vi "Make.vi"(8 "error in (no error)":errorcluster, 11 "Electrical in":refnum<class "Electrical.lvclass">) -> (0 "error out":errorcluster, 3 "Electrical out":refnum<class "Electrical.lvclass">)   [LabVIEW 2014, in "Electrical.lvclass"]
uses:
  Electrical.lvclass
  Paint/Paint.lvclass
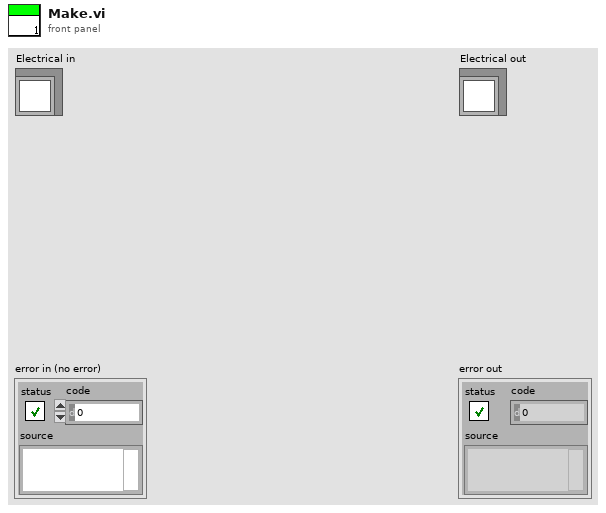
[diagram p1: front panel]
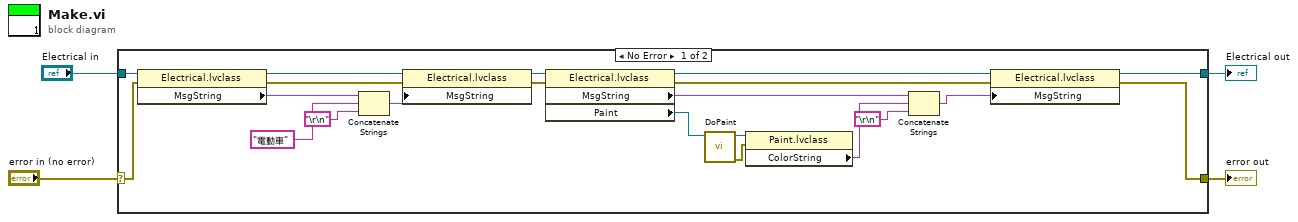
[diagram p0: block diagram]
diagram:
  n1 = case shown="No Error" "error in (no error)" {
    selector: "error in (no error)" -> [w25 w27]
    tunnel: [w8 w27] -> w4
    tunnel: [w6 w26] -> w3
    tunnel: "Electrical in" -> [w23 w26]
    frame No Error {
      n2 = property class="Electrical.lvclass"(reference=w23, error in=w25) -> (reference out=w21:refnum<class "Electrical.lvclass">, error out=w24:errorcluster, "MsgString"=w20:string)
      n3 = Concatenate Strings(w20, "電動車", "\r\n") -> (w19:string)
      n4 = property class="Electrical.lvclass"(reference=w21, error in=w24, "MsgString"=w19) -> (reference out=w15:refnum<class "Electrical.lvclass">, error out=w22:errorcluster)
      n5 = property class="Electrical.lvclass"(reference=w15, error in=w22) -> (reference out=w7:refnum<class "Electrical.lvclass">, error out=w16:errorcluster, "MsgString"=w10:string, "Paint"=w12:refnum<class "Paint.lvclass">)
      n6 = call-dynamic "DoPaint.vi"("Paint in"=w12) -> ("error out"=w13:errorcluster, "Paint out"=w14:refnum<class "Paint.lvclass">)  [unwired: 9 in]
      n7 = property class="Paint.lvclass"(reference=w14, error in=w13) -> ("ColorString"=w9:string)  [unwired: 2 out]
      n8 = Concatenate Strings(w10, w9, "\r\n") -> (w5:string)
      n9 = property class="Electrical.lvclass"(reference=w7, error in=w16, "MsgString"=w5) -> (reference out=w6:refnum<class "Electrical.lvclass">, error out=w8:errorcluster)
    }
    frame Error {
    }
  }
  "error out" <- w4
  "Electrical out" <- w3
